vi "CustomEventHandler.vi"(11 "MicronGRPC.lvclass":refnum<class "MicronGRPC.lvclass">) -> ()   [LabVIEW 2019, in "MicronGRPCGeneratedServer.lvlib"]
uses:
  MicronGRPCGeneratedServer.lvlib
  RPC Service/MicronGRPC/MicronGRPC.lvclass
  Message/GRPCMessage.lvclass
  D:/GitHub/KarthikAbiram/Micron/Source/Base/Server/Message/MessageBase.lvclass
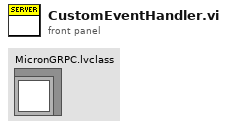
[diagram p1: front panel]
types:
  T1 = typedef "grpc-lvsupport-release.lvlib/grpcId.ctl" = u64
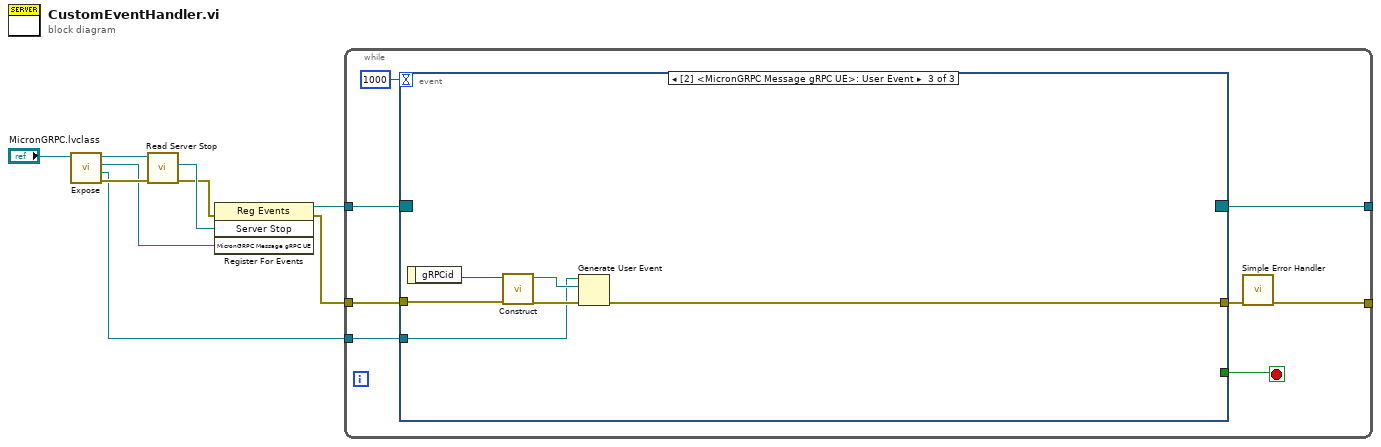
[diagram p0: block diagram]
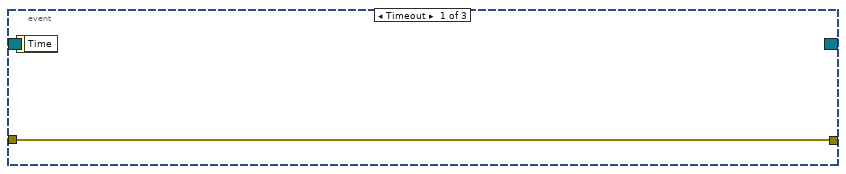
[diagram p2: hidden frame]
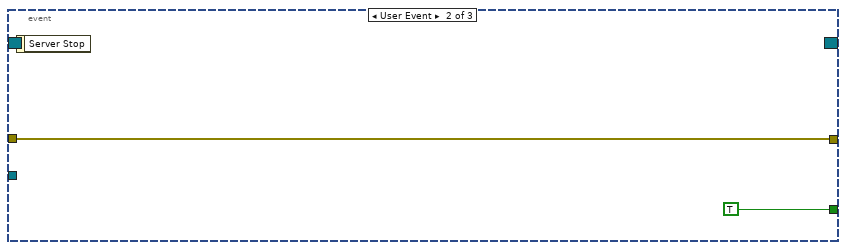
[diagram p3: hidden frame]
diagram:
  n1 = call "Expose.vi"("MicronGRPC in"="MicronGRPC.lvclass") -> ("error out"=w4:errorcluster, "MicronUE"=w1:refnum<user-event>, "MicronGRPC Message gRPC UE"=w3:refnum<user-event>, "MicronGRPC out"=w5:refnum<class "MicronGRPC.lvclass">)  [unwired: 7 in]
  n2 = call-dynamic "Read Server Stop.vi"("error in"=w4, "iService in"=w5) -> ("error out"=w2:errorcluster, "Server Stop"=w9:refnum<user-event>)  [unwired: 7 in, 1 out]
  n3 = register-events(error in=w2, w9, w3) -> (reference out=w8:refnum<event-registration>, error out=w7:errorcluster)  [unwired: 1 in]
  n4 = while {
    tunnel: w8 -> [w17]
    tunnel: [w15] -> _
    tunnel: w7 -> [w13]
    tunnel: [w11] -> _
    tunnel: w1 -> [w10]
    stop <- w16 stop-if-true
    n5 = event "RPC Methods Event Structure" shown="[2] <MicronGRPC Message gRPC UE>: User Event" {
      selector: w17 -> [_ _ _]
      dyn-events: [_ _ _] -> w15
      timeout: 1000 -> [_ _ _]
      tunnel: [_ TRUE _] -> w16
      tunnel: w13 -> [w18 w19 w23]
      tunnel: [w18 w19 w22] -> w12
      tunnel: w10 -> [_ _ w21]
      event Timeout {
        n6 = event-data() -> ()  [unwired: 1 in, 1 out]
      }
      event User Event {
        n7 = event-data() -> ()  [unwired: 1 in, 1 out]
      }
      event User Event {
        n8 = event-data() -> ("gRPCid"=w26:T1)  [unwired: 1 in]
        n9 = call "Construct.vi"("error in (no error)"=w23, "gRPCid"=w26) -> ("error out"=w25:errorcluster, "GRPCMessage out"=w24:refnum<class "GRPCMessage.lvclass">)  [unwired: 8 in]
        n10 = Generate User Event(user event=w21, event data cluster=w24, error in=w25) -> (error out=w22:errorcluster)  [unwired: 1 in, 1 out]
      }
    }
    n11 = call <vilib>:"Simple Error Handler.vi"("error in (no error)"=w12) -> ("error out"=w11:errorcluster)  [unwired: 4 in, 4 out]
  }
